vi "ParameterInterceptorType.vi"(0 "Data name":string) -> (1 "Array level":i32, 2 "Interceptor style":string)   [LabVIEW 2013]
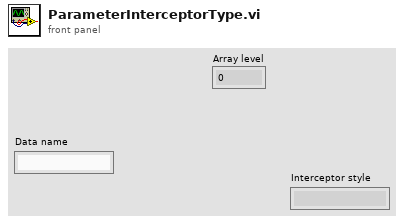
[diagram p1: front panel]
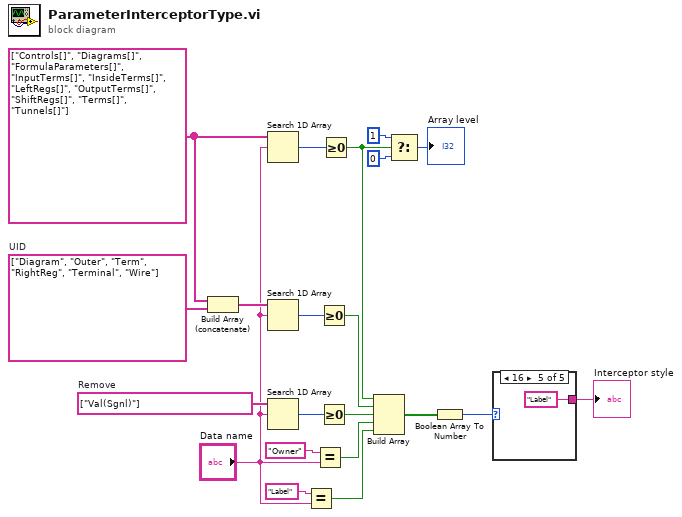
[diagram p0: block diagram]
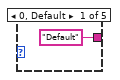
[diagram p2: hidden frame]
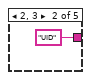
[diagram p3: hidden frame]
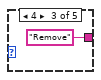
[diagram p4: hidden frame]
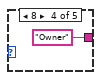
[diagram p5: hidden frame]
diagram:
  w10 = string[] ["Val(Sgnl)"]  # Remove
  w7 = string[] ["Diagram", "Outer", "Term", "RightReg", "Terminal", "Wire"]  # UID
  w8 = string[] ["Controls[]", "Diagrams[]", "FormulaParameters[]", "InputTerms[]", "InsideTerms[]", "LeftRegs[]", "OutputTerms[]", "ShiftRegs[]", "Terms[]", "Tunnels[]"]
  n1 = Build Array (concatenate)(w8, w7) -> (w6:string[])
  n2 = Search 1D Array(1D array=w8, element="Data name") -> (index of element=w21:i32)  [unwired: 1 in]
  n3 = Search 1D Array(1D array=w6, element="Data name") -> (index of element=w17:i32)  [unwired: 1 in]
  n4 = Search 1D Array(1D array=w10, element="Data name") -> (index of element=w11:i32)  [unwired: 1 in]
  n5 = Equal?(x="Label" ("Remove"), y="Data name") -> (x = y?=w1:bool)
  n6 = Equal?(x="Owner" ("Remove"), y="Data name") -> (x = y?=w4:bool)
  n7 = Greater Or Equal To 0?(x=w17) -> (x >= 0?=w15:bool)
  n8 = Greater Or Equal To 0?(x=w11) -> (x >= 0?=w9:bool)
  n9 = Greater Or Equal To 0?(x=w21) -> (x >= 0?=w16:bool)
  n10 = Build Array(w16, w15, w9, w4, w1) -> (w14:bool[])
  n11 = Select(t=1, s=w16, f=0) -> (s? t:f=→"Array level":i32)
  n12 = Boolean Array To Number(Boolean array=w14) -> (number=w13:u32)
  n13 = case shown="16" w13 {
    tunnel: ["Default" "UID" "Remove" "Owner" "Label"] -> w12
    frame 0, Default {
    }
    frame 2, 3 {
    }
    frame 4 {
    }
    frame 8 {
    }
    frame 16 {
    }
  }
  "Interceptor style" <- w12
